vi "Publish Group.vi"(8 "error in (no error)":errorcluster, 10 "Group":refnum<class "GroupAbstract.lvclass">, 11 "Task in":refnum<class "Task.lvclass">) -> (0 "error out":errorcluster, 3 "Task out":refnum<class "Task.lvclass">)   [LabVIEW 2020, in "Volatus.lvlib" / "Task.lvclass"]
uses:
  Task.lvclass
  Task.lvclass/Task.ctl
  TelemetryAPI/TelemetryAPI.lvclass
  lv-vecto/Vecto/GroupAbstract/GroupAbstract.lvclass
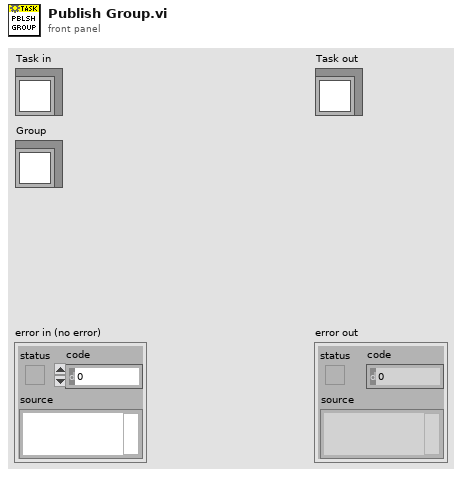
[diagram p1: front panel]
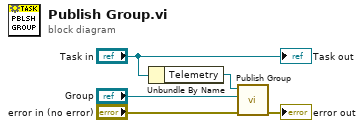
[diagram p0: block diagram]
diagram:
  n1 = Unbundle By Name("Task in") -> ("Telemetry"=w4:refnum<class "TelemetryAPI.lvclass">)
  n2 = call "Publish Group.vi"("error in (no error)"="error in (no error)", "Group"="Group", "TelemetryAPI in"=w4) -> ("error out"=→"error out":errorcluster)  [unwired: 7 in, 1 out]
  "Task out" <- "Task in"
